vi "DrawTopMenu.vi"(8 "error in (no error)":errorcluster, 10 "Coords":T2, 11 "Menu in":refnum<class "Menu.lvclass">) -> (0 "error out":errorcluster, 1 "Selected Tag":string, 2 "Selected Area":T1, 3 "Menu out":refnum<class "Menu.lvclass">, 4 "SubMenu":bool)   [LabVIEW 2021, in "Menu.lvlib" / "Menu.lvclass"]
uses:
  Menu.lvclass
  Menu.lvclass/Menu.ctl
  Picture2D/src/Collection/Collection.lvclass
  Picture2D/src/2DPictureControl/2DPictureControl.lvclass
  C:/GitHub/Picture2D/src/Picture2D/Picture2D.lvclass
  C:/GitHub/Picture2D/src/IDrawable/IDrawable.lvclass
  C:/GitHub/Picture2D/src/IMovable/IMovable.lvclass
  C:/GitHub/Picture2D/src/IRotatable/IRotatable.lvclass
  C:/GitHub/Picture2D/src/IScalable/IScalable.lvclass
  C:/GitHub/Picture2D/src/Collection/Collection.lvclass
  <vilib>/Utility/miscctls.llb/LVPoint32TypeDef.ctl
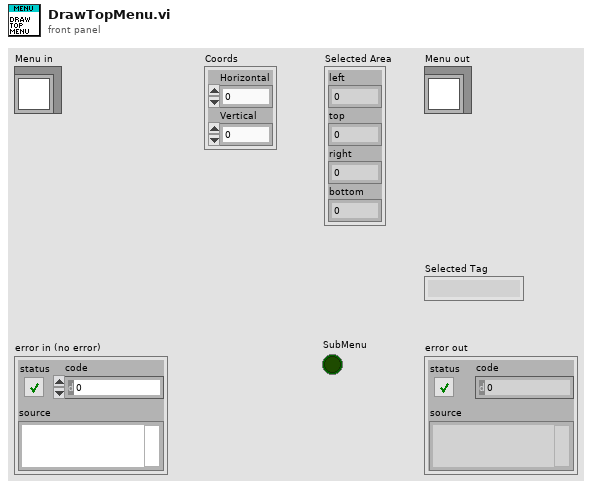
[diagram p1: front panel]
types:
  T1 = cluster{"left":i16, "top":i16, "right":i16, "bottom":i16}
  T2 = typedef "LVPoint32TypeDef.ctl" = cluster{"Horizontal":i32, "Vertical":i32}
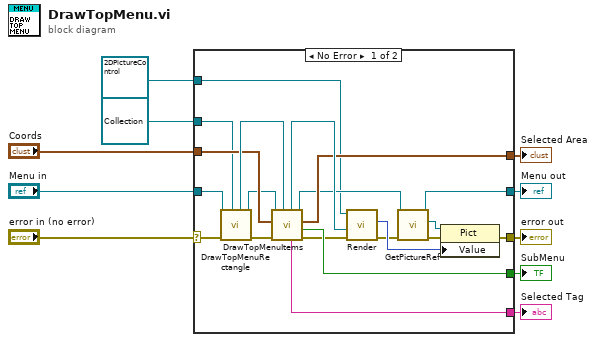
[diagram p0: block diagram]
diagram:
  n1 = case shown="No Error" "error in (no error)" {
    selector: "error in (no error)" -> [w21 w31]
    tunnel: [w28 _] -> w10
    tunnel: [w27 _] -> w9
    tunnel: [w26 w31] -> w8
    tunnel: [w25 _] -> w7
    tunnel: "Coords" -> [w22 _]
    tunnel: [w16 w32] -> w4
    tunnel: "Menu in" -> [w13 w32]
    tunnel: refnum<class "Collection.lvclass"> refnum ("Picture2D.lvlib:Collection.lvclass") -> [w12 _]
    tunnel: refnum<class "2DPictureControl.lvclass"> refnum ("2DPictureControl in") -> [w11 _]
    frame No Error {
      n2 = call "DrawTopMenuRectangle.vi"("Collection in"=w12, "error in (no error)"=w21, "Menu in"=w13) -> ("error out"=w20:errorcluster, "Menu out"=w19:refnum<class "Menu.lvclass">, "Collection out"=w23:refnum<class "Collection.lvclass">)  [unwired: 6 in]
      n3 = call "DrawTopMenuItems.vi"("Collection in"=w23, "error in (no error)"=w20, "Coords"=w22, "Menu in"=w19) -> ("error out"=w24:errorcluster, "SubMenu"=w25:bool, "Area out"=w27:T1, "Menu out"=w17:refnum<class "Menu.lvclass">, "SelectedItemTeg"=w28:string, "Collection out"=w29:refnum<class "Collection.lvclass">)  [unwired: 2 in]
      n4 = call-dynamic "Render.vi"("error in (no error)"=w24, "IDrawable"=w29, "2DPictureControl in"=w11) -> ("error out"=w14:errorcluster, "2D Picture out"=w30:picture)  [unwired: 6 in, 1 out]
      n5 = call "GetPictureRef.vi"("error in (no error)"=w14, "Menu in"=w17) -> ("error out"=w15:errorcluster, "PictRef"=w18:refnum<vi>, "Menu out"=w16:refnum<class "Menu.lvclass">)  [unwired: 7 in]
      n6 = property class="Pict"(reference=w18, error in=w15, "Value"=w30) -> (error out=w26:errorcluster)  [unwired: 1 out]
    }
    frame Error {
    }
  }
  "Selected Tag" <- w10
  "Selected Area" <- w9
  "error out" <- w8
  "Menu out" <- w4
  "SubMenu" <- w7
